vi "Pump Runtime Calc.vi"(1 "RPM":i32, 2 "Accel":i32=50, 3 "Strokes":i32) -> (0 "Pump Runtime (s)":dbl)   [LabVIEW 2019]
panel:
  out "radians":dbl
  out "rad/s":dbl
  out "time at set speed":dbl
  out "rad at set rpm":dbl
  out "rad during ramp":dbl
  out "ramp (s)":dbl
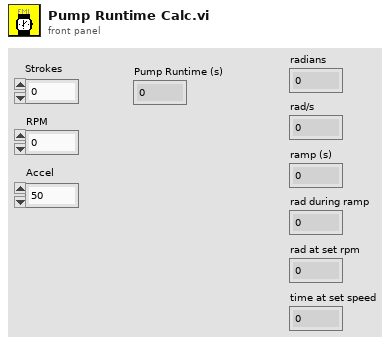
[diagram p1: front panel]
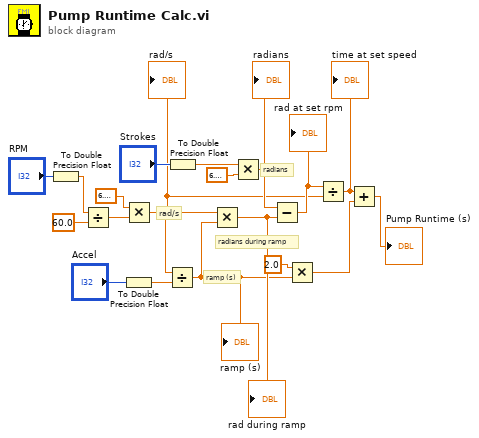
[diagram p0: block diagram]
diagram:
  # "radians"
  # "radians during ramp"
  # "rad/s"
  # "ramp (s)"
  n1 = To Double Precision Float(number="RPM") -> (double precision float=w2:dbl)
  n2 = Divide(x=w2, y=60.0) -> (x/y=w14:dbl)
  n3 = Multiply(x=6.283185307179586, y=w14) -> (x*y=w3:dbl)
  "rad/s" <- w3
  n4 = To Double Precision Float(number="Accel") -> (double precision float=w12:dbl)
  n5 = Divide(x=w3, y=w12) -> (x/y=w8:dbl)
  "ramp (s)" <- w8
  n6 = To Double Precision Float(number="Strokes") -> (double precision float=w19:dbl)
  n7 = Multiply(x=w3, y=w8) -> (x*y=w10:dbl)
  "rad during ramp" <- w10
  n8 = Multiply(x=w19, y=6.283185307179586) -> (x*y=w11:dbl)
  "radians" <- w11
  n9 = Subtract(x=w11, y=w10) -> (x-y=w4:dbl)
  "rad at set rpm" <- w4
  n10 = Multiply(x=2.0, y=w8) -> (x*y=w7:dbl)
  n11 = Divide(x=w4, y=w3) -> (x/y=w9:dbl)
  "time at set speed" <- w9
  n12 = Add(x=w9, y=w7) -> (x+y=→"Pump Runtime (s)":dbl)
